vi "analog i enkoder-synchronizacja.vi"() -> ()   [LabVIEW 2013]
uses:
  Kontrolki/KartaDAQ/ACQ all read tasks.ctl
  Kontrolki/KartaDAQ/ACQ analog channel config new.ctl
  Kontrolki/KartaDAQ/ACQ counter channel config.ctl
  <vilib>/Utility/error.llb/DialogType.ctl
  <vilib>/DAQmx/configure/task.llb/DAQmx Start Task.vi
  <vilib>/Waveform/WDTOps.llb/WDT Append Waveforms DBL.vi
panel:
  out "Array":u32[](array[numeric])
  out "loop delay":u32
  out "Iteracja":i32
  out "Waveform Graph":waveform(dbl)[](graph)
  in  "stop":bool
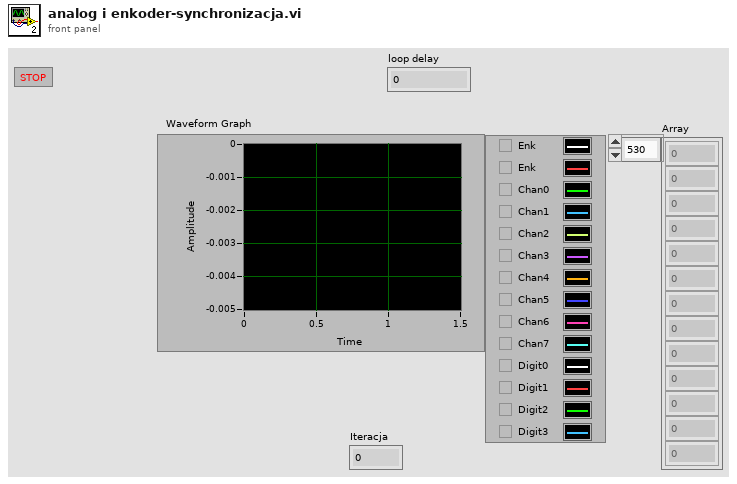
[diagram p1: front panel]
types:
  T1 = typedef "DialogType.ctl" = u16
  T2 = typedef "ACQ counter channel config.ctl" = cluster{"Enkoder X":string, "Enkoder Y":string, "Generator":string, "Generator OUT":string}
  T3 = typedef "ACQ analog channel config new.ctl" = cluster{"Analogs IN":string[], "Digitals IN":string[]}
  T4 = typedef "ACQ all read tasks.ctl" = cluster{"Enkoder X ref":refnum<k21>, "Enkoder Y ref":refnum<k21>, "Generator ref":refnum<k21>, "Analog ref":refnum<k21>}
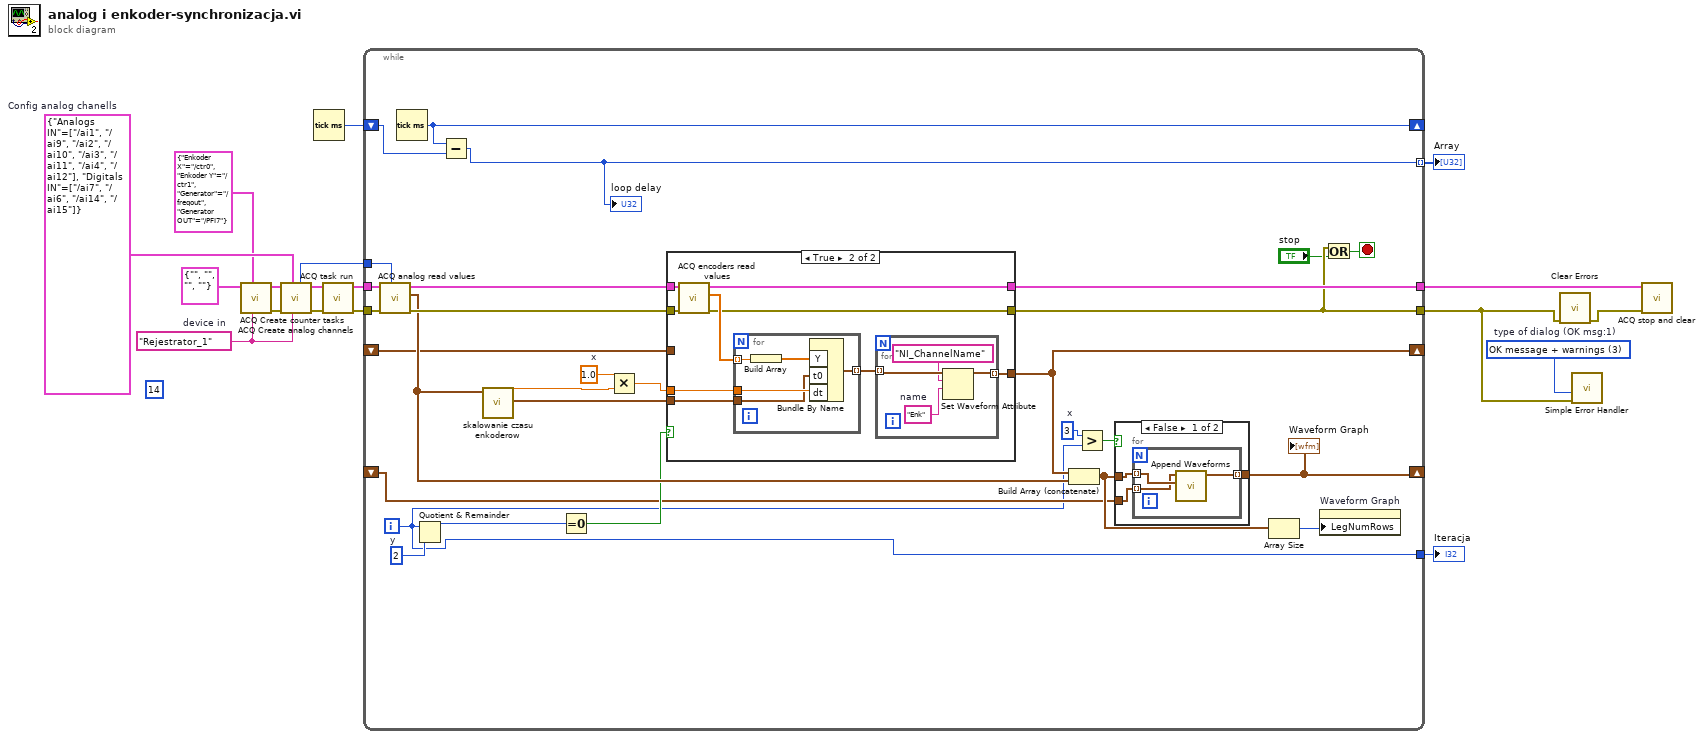
[diagram p0: block diagram]
diagram:
  (unwired) 14
  w5 = T1 3 items=["no dialog", "OK message", "continue or stop message", "OK message + warnings", "continue/stop + warnings"]  # type of dialog (OK msg:1)
  w12 = tag "Rejestrator_1"  # device in
  w13 = T3 {"Analogs IN"=["/ai1", "/ai9", "/ai2", "/ai10", "/ai3", "/ai11", "/ai4", "/ai12"], "Digitals IN"=["/ai7", "/ai6", "/ai14", "/ai15"]}  # Config analog chanells
  n1 = call "ACQ Create counter tasks.vi"("device in"=w12, "Config Counter channels"=T2 {"Enkoder X"="/ctr0", "Enkoder Y"="/ctr1", "Generator"="/freqout", "Generator OUT"="/PFI7"}, "All Read tasks in"=T4 {"Enkoder X ref"="", "Enkoder Y ref"="", "Generator ref"="", "Analog ref"=""}) -> ("error out"=w18:errorcluster, "All Read tasks out"=w14:T4)  [unwired: 6 in, 1 out]
  n2 = call "ACQ Create analog channels.vi"("device in"=w12, "Config analog chanells new"=w13, "error in (no error)"=w18, "All Read tasks in"=w14) -> ("error out"=w17:errorcluster, "All Read tasks out"=w15:T4, "samples per channel"=w7:i32)  [unwired: 4 in, 1 out]
  n3 = Tick Count (ms)() -> (millisecond timer value=w6:u32)
  n4 = call "ACQ task run.vi"("error in (no error)"=w17, "All Read tasks in"=w15) -> ("error out"=w9:errorcluster, "All Read tasks out"=w10:T4)  [unwired: 7 in, 1 out]
  n5 = while {
    tunnel: w10 -> [w47]
    tunnel: w9 -> [w46]
    tunnel: [w35] -> w3
    tunnel: [w43] -> w8
    tunnel: w7 -> [w42]
    shift-right: [w40] -> _
    shift-left: w6 -> [w41]
    shift-right: [w29] -> _
    shift-left: _ -> [w28]
    tunnel: [w22] -> w2
    tunnel: [w27] -> w1 mode=indexing
    shift-right: [w25] -> _
    shift-left: _ -> [w24]
    i -> [w22]
    stop <- w36 stop-if-true
    w21 = 3  # x
    w32 = 2  # y
    w33 = 1.0  # x
    n6 = call "ACQ analog read values.vi"("samples per channel"=w42, "error in (no error)"=w46, "Tasks ref in"=w47) -> ("error out"=w44:errorcluster, "data"=w37:waveform(dbl)[], "Tasks ref out"=w45:T4)  [unwired: 6 in]
    n7 = Tick Count (ms)() -> (millisecond timer value=w40:u32)
    n8 = Quotient & Remainder(x=w22, y=w32) -> (x-y*floor(x/y)=w31:i32)  [unwired: 1 out]
    n9 = Subtract(x=w40, y=w41) -> (x-y=w27:u32)
    "loop delay" <- w27
    n10 = call "skalowanie czasu enkoderow.vi"("data"=w37) -> ("t0"=w39:timestamp, "dT out"=w19:dbl)  [unwired: 9 in]
    n11 = Equal To 0?(x=w31) -> (x = 0?=w30:bool)
    n12 = Multiply(x=w33, y=w19) -> (x*y=w20:dbl)
    n13 = case shown="True" w30 {
      tunnel: w45 -> [w57 w66]
      tunnel: w44 -> [w56 w65]
      tunnel: [w57 w64] -> w43
      tunnel: w39 -> [_ w62]
      tunnel: [w55 w60] -> w29
      tunnel: [w56 w59] -> w35
      tunnel: w20 -> [_ w58]
      tunnel: w28 -> [w55 _]
      frame False {
      }
      frame True {
        n14 = call "ACQ encoders read values.vi"("error in (no error)"=w65, "Tasks ref in"=w66) -> ("error out"=w59:errorcluster, "Encoders out"=w63:dbl[], "Tasks ref out"=w64:T4)  [unwired: 7 in]
        n15 = for {
          tunnel: w63 -> [w75] mode=indexing
          tunnel: w58 -> [w73]
          tunnel: w62 -> [w72]
          tunnel: [w71] -> w61 mode=indexing
          n16 = Build Array(w75) -> (w74:dbl[])
          n17 = Bundle By Name("Y"=w74, "t0"=w72, "dt"=w73) -> (w71:waveform(dbl))  [unwired: 1 in]
        }
        n18 = for {
          tunnel: w61 -> [w70] mode=indexing
          tunnel: [w69] -> w60 mode=indexing
          w67 = "Enk"  # name
          n19 = Set Waveform Attribute(5:w67, 6:"NI_ChannelName" ("name"), 7:w70) -> (3:w69:waveform(dbl))  [unwired: 1 in, 2 out]
        }
      }
    }
    n20 = Build Array (concatenate)(w29, w37) -> (w26:waveform(dbl)[])
    n21 = Greater?(x=w21, y=w22) -> (0:w23:bool)
    n22 = case shown="False" w23 {
      tunnel: w26 -> [w50 w54]
      tunnel: [w49 w54] -> w25
      tunnel: w24 -> [w48 _]
      frame False {
        n23 = for {
          tunnel: w50 -> [w53] mode=indexing
          tunnel: [w52] -> w49 mode=indexing
          tunnel: w48 -> [w51] mode=indexing
          n24 = call-poly <vilib>:"Append Waveforms.vi"("waveform B"=w53, "waveform A"=w51) -> ("waveform out"=w52:waveform(dbl))  [unwired: 8 in, 1 out]
        }
      }
      frame True {
      }
    }
    "Waveform Graph" <- w25
    n25 = Array Size(array=w26) -> (size(s)=w38:i32)
    n26 = property on="Waveform Graph" class="WFGraph (strict)"("LegNumRows"=w38) -> ()  [unwired: 2 in, 2 out]
    n27 = Or(x=w35, y="stop") -> (x .or. y?=w36:bool)
  }
  "Iteracja" <- w2
  "Array" <- w1
  n28 = call <vilib>:"Clear Errors.vi"("error in (no error)"=w3) -> ("error out"=w4:errorcluster)  [unwired: 6 in]
  n29 = call <vilib>:"Simple Error Handler.vi"("type of dialog (OK msg:1)"=w5, "error in (no error)"=w3) -> ()  [unwired: 3 in, 5 out]
  n30 = call "ACQ stop and clear.vi"("error in (no error)"=w4, "Tasks ref in"=w8) -> ()  [unwired: 9 in, 1 out]
